vi "Multiply Numbers.vi"(8 "error in (no error)":errorcluster, 9 "Number 2":dbl, 10 "Number 1":dbl, 11 "Multiplication Actor in":refnum<class "Multiplication Actor.lvclass">) -> (0 "error out":errorcluster, 3 "Multiplication Actor out":refnum<class "Multiplication Actor.lvclass">)   [LabVIEW 2014, in "Multiplication Actor.lvclass"]
uses:
  Multiplication Actor.lvclass
  <vilib>/ActorFramework/Actor/Actor.lvclass/Actor.ctl
  <vilib>/ActorFramework/Actor/Actor.lvclass
  Calculator Actor/Calculator Actor Messages/Multiplication Result Msg/Multiplication Result Msg.lvclass
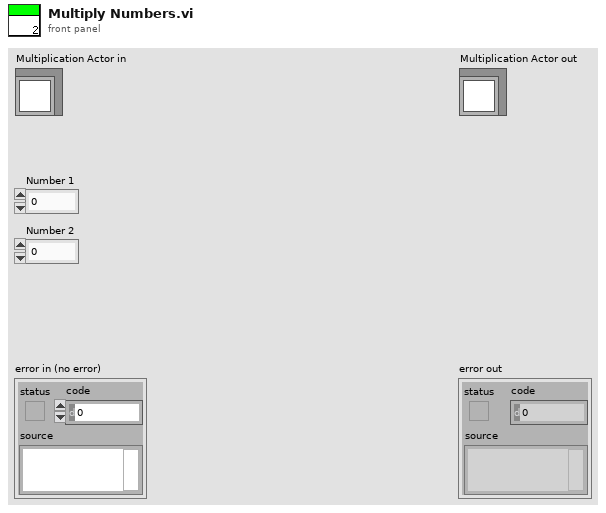
[diagram p1: front panel]
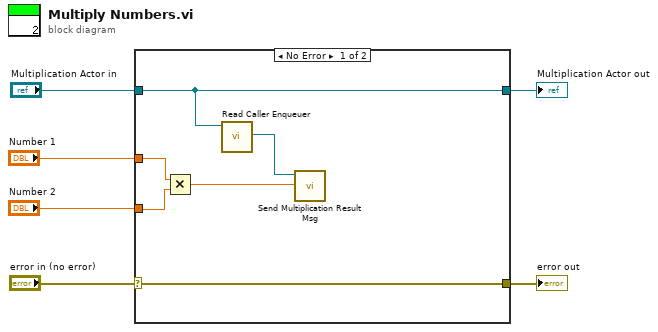
[diagram p0: block diagram]
diagram:
  n1 = case shown="No Error" "error in (no error)" {
    selector: "error in (no error)" -> [w12 w14]
    tunnel: [w12 w14] -> w5
    tunnel: [w9 w13] -> w3
    tunnel: "Multiplication Actor in" -> [w9 w13]
    tunnel: "Number 1" -> [w11 _]
    tunnel: "Number 2" -> [w10 _]
    frame No Error {
      n2 = Multiply(x=w11, y=w10) -> (x*y=w8:dbl)
      n3 = call <vilib>:"Read Caller Enqueuer.vi"("Actor"=w9) -> ("Caller Enqueuer"=w7:refnum<class "Message Enqueuer.lvclass">)  [unwired: 10 in]
      n4 = call "Send Multiplication Result Msg.vi"("Multiplication Result"=w8, "Message Enqueuer in"=w7) -> ()  [unwired: 8 in, 2 out]
    }
    frame Error {
    }
  }
  "error out" <- w5
  "Multiplication Actor out" <- w3
